vi "IntensityToRGBScale.vi"(1 "Threshold (max)":u32, 2 "Intensity":u32[][](array[numeric])) -> (0 "RGB Scale":u32[][](array[numeric]))   [LabVIEW 2009]
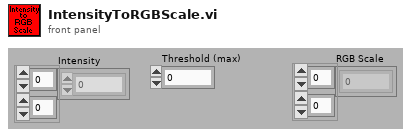
[diagram p1: front panel]
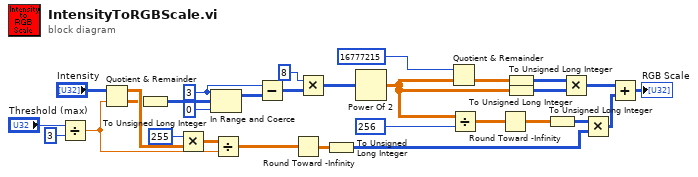
[diagram p0: block diagram]
diagram:
  w16 = 3
  n1 = Divide(x="Threshold (max)", y=u32 3) -> (x/y=w5:dbl)
  n2 = Quotient & Remainder(x="Intensity", y=w5) -> (x-y*floor(x/y)=w25:dbl[][], floor(x/y)=w12:dbl[][])
  n3 = To Unsigned Long Integer(number=w12) -> (unsigned 32bit integer=w20:u32[][])
  n4 = Multiply(x=u32 255, y=w25) -> (x*y=w6:dbl[][])
  n5 = In Range and Coerce(upper limit=w16, x=w20, lower limit=0) -> (coerced(x)=w15:u32[][])  [unwired: 1 out]
  n6 = Divide(x=w6, y=w5) -> (x/y=w4:dbl[][])
  n7 = Subtract(x=w16, y=w15) -> (x-y=w17:u32[][])
  n8 = Round Toward -Infinity(1:w4) -> (0:w26:dbl[][])
  n9 = Multiply(x=8, y=w17) -> (x*y=w19:u32[][])
  n10 = To Unsigned Long Integer(number=w26) -> (unsigned 32bit integer=w28:u32[][])
  n11 = Power Of 2(x=w19) -> (2^x=w8:dbl[][])
  n12 = Quotient & Remainder(x=u32 16777215, y=w8) -> (floor(x/y)=w7:dbl[][])  [unwired: 1 out]
  n13 = Divide(x=w8, y=u32 256) -> (x/y=w27:dbl[][])
  n14 = Round Toward -Infinity(1:w27) -> (0:w29:dbl[][])
  n15 = To Unsigned Long Integer(number=w7) -> (unsigned 32bit integer=w21:u32[][])
  n16 = To Unsigned Long Integer(number=w8) -> (unsigned 32bit integer=w22:u32[][])
  n17 = To Unsigned Long Integer(number=w29) -> (unsigned 32bit integer=w30:u32[][])
  n18 = Multiply(x=w21, y=w22) -> (x*y=w1:u32[][])
  n19 = Multiply(x=w30, y=w28) -> (x*y=w3:u32[][])
  n20 = Add(x=w1, y=w3) -> (x+y=→"RGB Scale":u32[][])
